vi "RCM Show Block Diagram MHLC.vi"(8 "error in (no error)":errorcluster, 10 "Tree RCM Data":T1, 11 "AppMgr in":refnum<class "Application Manager.lvclass">) -> (0 "error out":errorcluster, 3 "AppMgr out":refnum<class "Application Manager.lvclass">)   [LabVIEW 2017, in "Application Manager.lvclass"]
doc: "Send Response Message to show the block diagram of the selected Worker's Main VI"
uses:
  Application Manager.lvclass
  Tree Right Click Menu Data.ctl
  <vilib>/Utility/miscctls.llb/LVPoint32TypeDef.ctl
  Application Manager.lvclass/Application Manager.ctl
  rsp_Show Worker Block Diagram.ctl
  Common VIs/DC_UID.ctl
  <vilib>/Utility/error.llb/Error Cluster From Error Code.vi
  <vilib>/ErrorRing/Error Ring.xnode
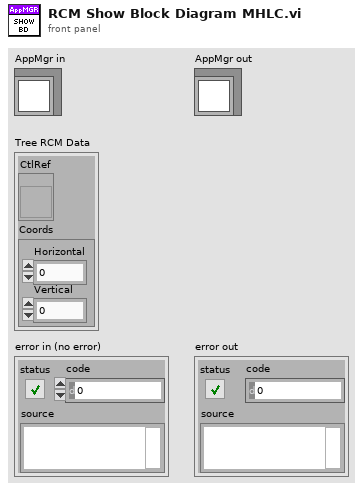
[diagram p1: front panel]
types:
  T1 = typedef "Application Manager.lvclass/Tree Right Click Menu Data.ctl" = cluster{"CtlRef":refnum<vi>, "Coords":T2}
  T2 = typedef "LVPoint32TypeDef.ctl" = cluster{"Horizontal":i32, "Vertical":i32}
  T3 = typedef "DC_UID.ctl" = string
  T4 = typedef "Application Manager.lvclass/Debug Client Data.ctl" = cluster{"DC_UID":T3, "IP Address":string, "Worker Data":T5[], "Connected":bool}
  T5 = typedef "Application Manager.lvclass/Worker Data.ctl" = cluster{"ID":string, "VI Ref":refnum<vi>, "VI Path":path, "CloneID":string, "Type":T6, "Worker Status":string}
  T6 = typedef "Workers.lvlib/Worker.lvclass/Worker Type.ctl" = enum16{"SL", "DL"}
  T7 = typedef "Application Manager.lvclass/rsp_Show Worker Block Diagram.ctl" = cluster{"DC_UID":T3, "VI Path":path, "VI Ref":refnum<vi>}
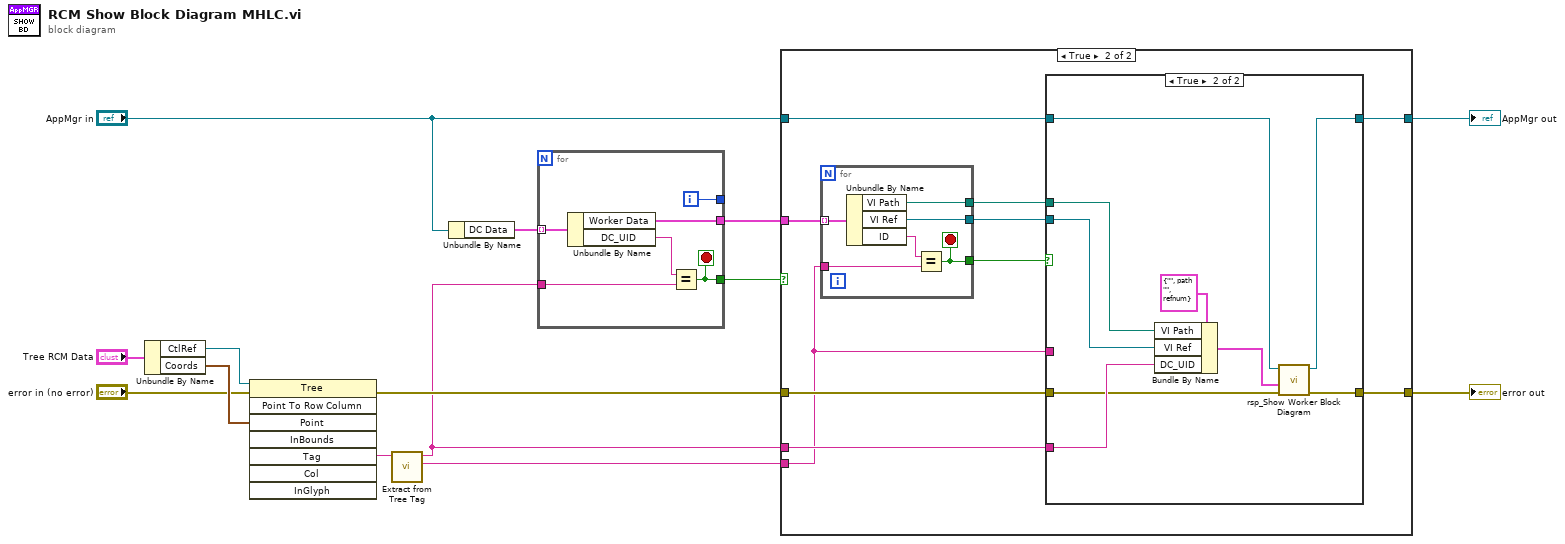
[diagram p0: block diagram]
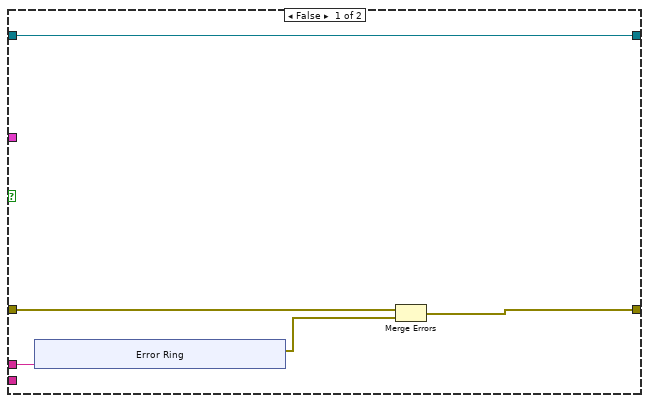
[diagram p2: hidden frame]
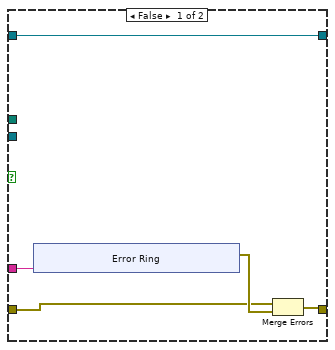
[diagram p3: hidden frame]
diagram:
  n1 = Unbundle By Name("Tree RCM Data") -> ("CtlRef"=w11:refnum<vi>, "Coords"=w10:T2)
  n2 = invoke class="Tree" method="Point To Row Column"(reference=w11, error in="error in (no error)", "Point"=w10) -> (error out=w9:errorcluster, "Tag"=w8:string)  [unwired: 5 in, 6 out]
  n3 = call "Extract from Tree Tag.vi"("Tag"=w8) -> ("WID"=w1:string, "DC_UID"=w7:T3)  [unwired: 9 in]
  n4 = Unbundle By Name("AppMgr in") -> ("DC Data"=w6:T4[])
  n5 = for {
    tunnel: w6 -> [w16] mode=indexing
    tunnel: [w19] -> w4
    tunnel: [w18] -> _
    tunnel: [w15] -> w5
    tunnel: w7 -> [w17]
    i -> [w18]
    stop <- w19 stop-if-true
    n6 = Unbundle By Name(w16) -> ("Worker Data"=w15:T5[], "DC_UID"=w20:T3)
    n7 = Equal?(x=w20, y=w17) -> (x = y?=w19:bool)
  }
  n8 = case shown="True" w4 {
    tunnel: [w24 w38] -> w12
    tunnel: w9 -> [w25 w39]
    tunnel: w7 -> [w22 w40]
    tunnel: w5 -> [_ w37]
    tunnel: "AppMgr in" -> [w21 w42]
    tunnel: [w21 w41] -> w13
    tunnel: w1 -> [_ w34]
    frame False {
      n9 = xnode "Error Ring"("parameter 0"=w22) -> ("error out"=w23:errorcluster)
      n10 = Merge Errors(w25, w23) -> (w24:errorcluster)
    }
    frame True {
      n11 = for {
        tunnel: w37 -> [w69] mode=indexing
        tunnel: w34 -> [w67]
        tunnel: [w66] -> w33
        tunnel: [w65] -> w35
        tunnel: [w64] -> w36
        stop <- w66 stop-if-true
        n12 = Unbundle By Name(w69) -> ("VI Path"=w65:path, "VI Ref"=w64:refnum<vi>, "ID"=w68:string)
        n13 = Equal?(x=w68, y=w67) -> (x = y?=w66:bool)
      }
      n14 = case shown="True" w33 {
        tunnel: w42 -> [w47 w61]
        tunnel: [w47 w60] -> w41
        tunnel: w40 -> [_ w59]
        tunnel: w39 -> [w45 w58]
        tunnel: [w43 w57] -> w38
        tunnel: w36 -> [_ w56]
        tunnel: w35 -> [_ w55]
        tunnel: w34 -> [w44 _]
        frame False {
          n15 = xnode "Error Ring"("parameter 0"=w44) -> ("error out"=w46:errorcluster)
          n16 = Merge Errors(w45, w46) -> (w43:errorcluster)
        }
        frame True {
          n17 = Bundle By Name(cluster=T7 {"DC_UID"="", "VI Path"=path "", "VI Ref"=refnum} ("Data in"), "VI Path"=w55, "VI Ref"=w56, "DC_UID"=w59) -> (w63:T7)
          n18 = call "rsp_Show Worker Block Diagram.vi"("error in"=w58, "Data in"=w63, "Application Manager in"=w61) -> ("error out"=w57:errorcluster, "dup Application Manager out"=w60:refnum<class "Application Manager.lvclass">)  [unwired: 7 in]
        }
      }
    }
  }
  "AppMgr out" <- w13
  "error out" <- w12
